vi "Pfeiffer-RVC300.ProcCases.vi"(0 "i ref in":refnum<vi>, 1 "selector":string, 2 "Data":T1, 3 "call cluster":T2={"Object"="", "Selector"="", "CallType"=enum."synchronous", "Async Object"="", "Async Selector"="", "Data Descriptor"="", "Data"=[], "Error #"=0, "Expire"=0}, 5 "error in (no error)":errorcluster) -> (14 "i ref out":refnum<vi>, 17 "answer cluster":T2={"Object"="", "Selector"="", "CallType"=enum."synchronous", "Async Object"="", "Async Selector"="", "Data Descriptor"="", "Data"=[], "Error #"=0, "Expire"=0}, 19 "error out":errorcluster)   [LabVIEW 2014, in "Pfeiffer-RVC300.lvlib"]
doc: "This method is called by a process from within the default case in the event loop. The methods of a class that are linked to events will be called from THIS method. Add your code here."
uses:
  Pfeiffer-RVC300.lvlib
  CS_Core/CSSystem/CoreDefs/CoreDefs.call_type.ctl
  CS_Core/BaseProcess/BaseProcess.descriptor string definition.ctl
  CS_Core/CSSystem/CoreDefs/CoreDefs.rawDataType.ctl
  CS_Core/CSSystem/CoreLib/CoreLib.byte array 2 double.vi
  CS_Core/CSSystem/CoreLib/CoreLib.double 2 byte array.vi
  CS_Core/CSSystem/CoreLib/CoreLib.string 2 byte array.vi
  CS_Core/CSSystem/CoreLib/CoreLib.byte array 2 int.vi
  CS_Core/CSSystem/CoreLib/CoreLib.lvlib
  CS_Core/BaseProcess/BaseProcess.lvlib
  CS_Core/CSApplicationBaseClasses/DeviceBase/DeviceBase.lvlib
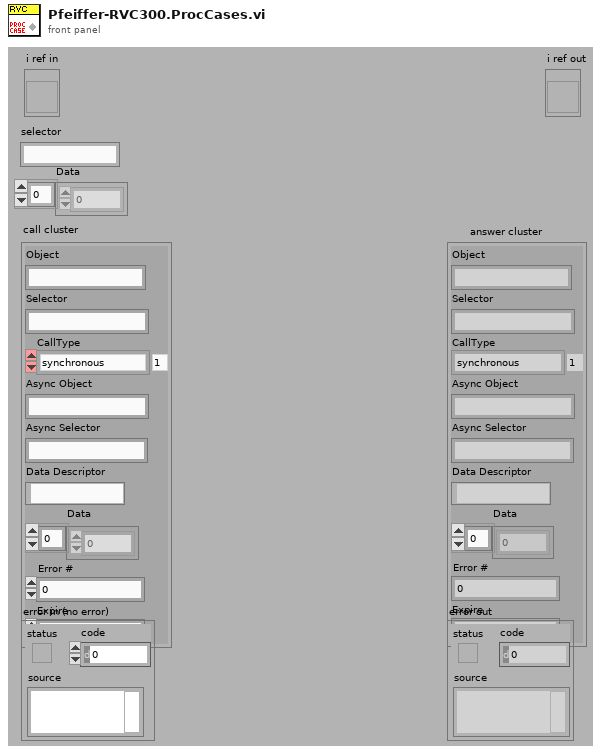
[diagram p1: front panel]
types:
  T1 = typedef "CoreDefs.rawDataType.ctl" = i8[]
  T2 = typedef "CoreDefs.call_type.ctl" = cluster{"Object":string, "Selector":string, "CallType":enum16{"simple", "synchronous", "asynchronous"}, "Async Object":string, "Async Selector":string, "Data Descriptor":T3, "Data":T1, "Error #":i32, "Expire":u32}
  T3 = typedef "BaseProcess.lvlib/BaseProcess.descriptor string definition.ctl" = string
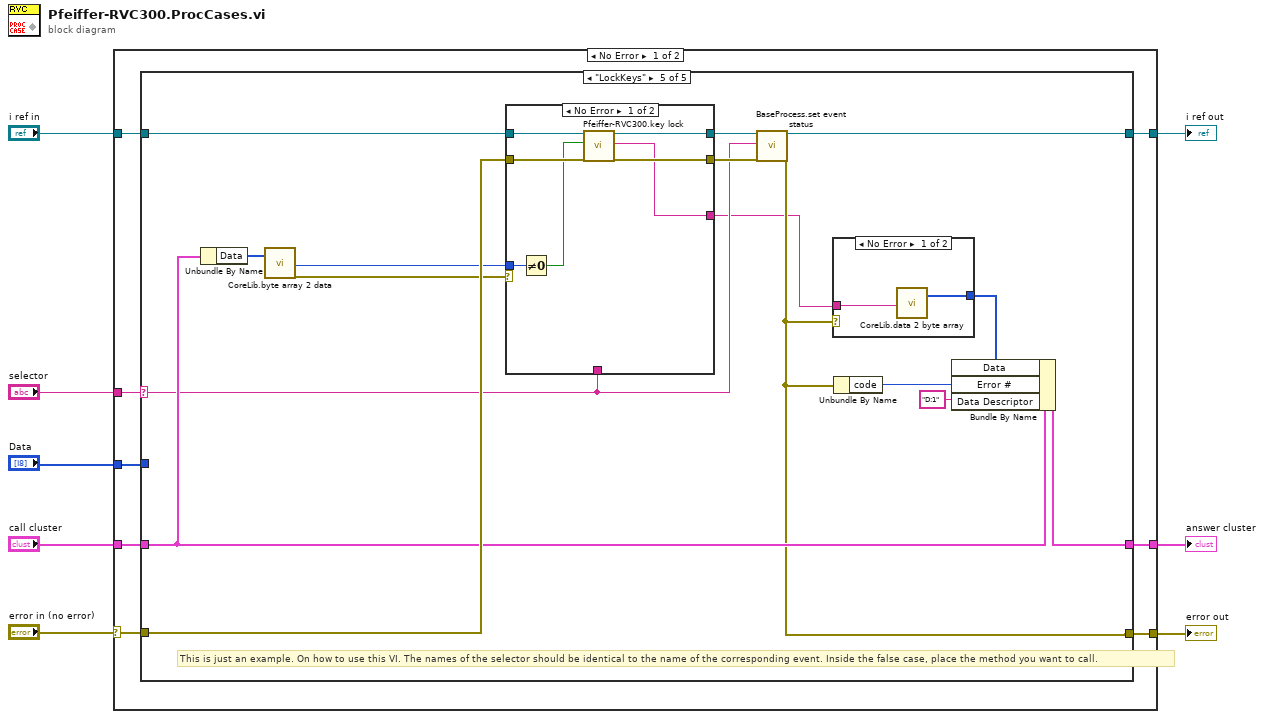
[diagram p0: block diagram]
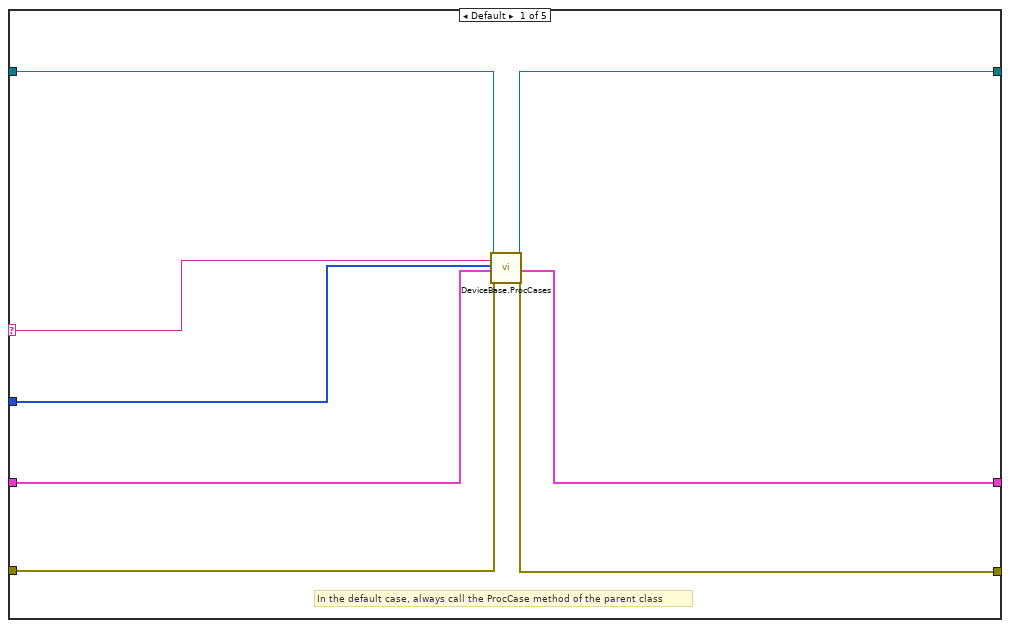
[diagram p2: hidden frame]
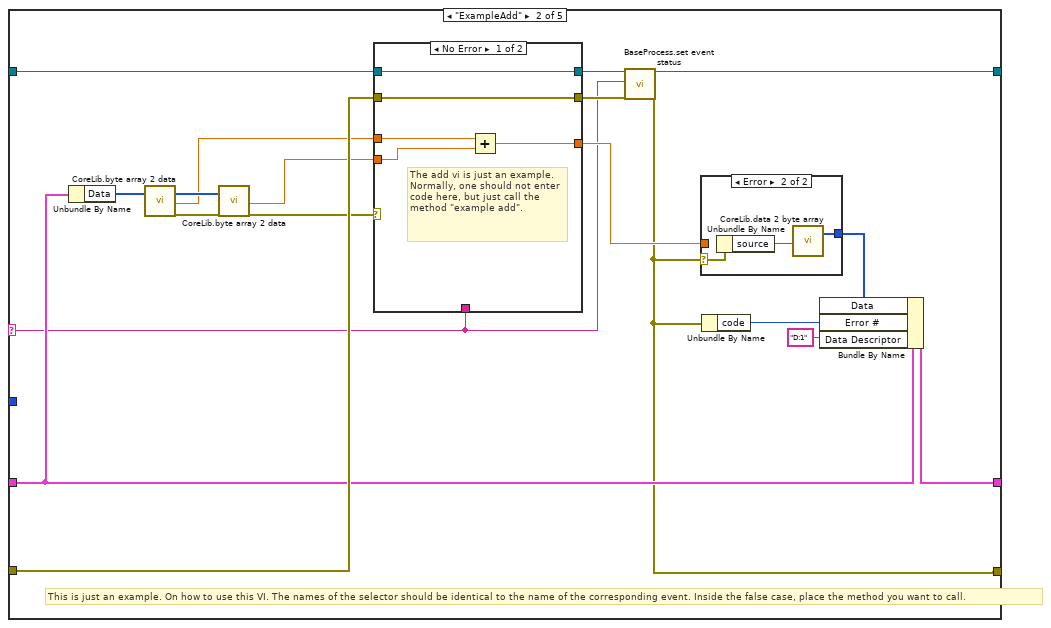
[diagram p3: hidden frame]
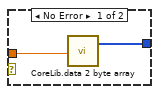
[diagram p4: hidden frame]
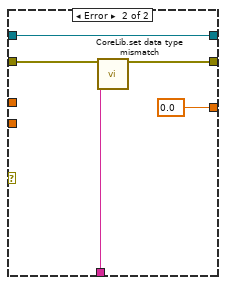
[diagram p5: hidden frame]
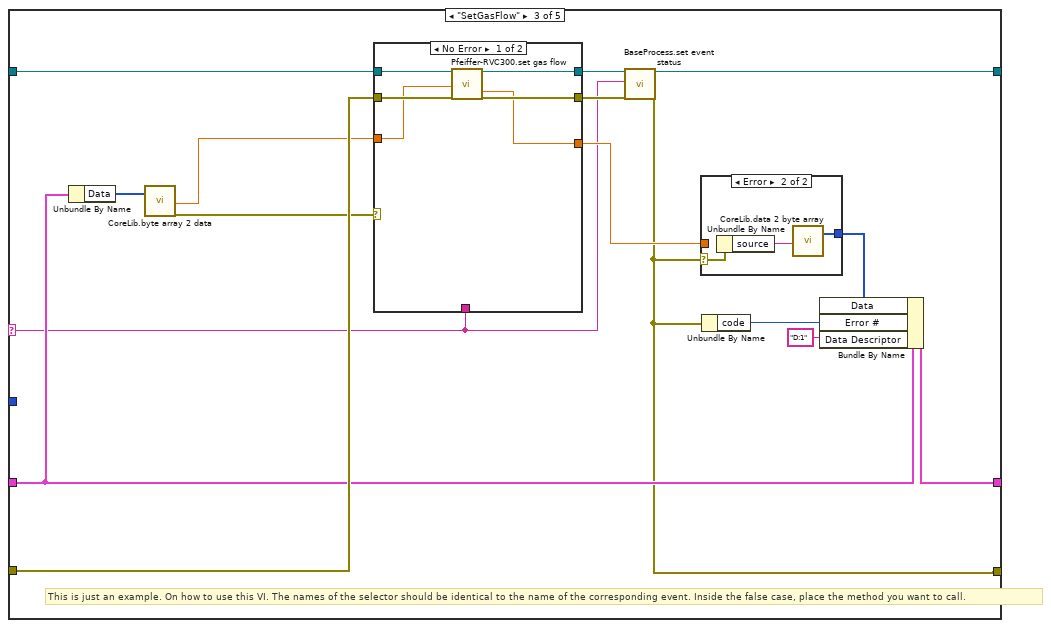
[diagram p6: hidden frame]
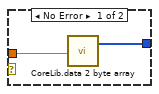
[diagram p7: hidden frame]
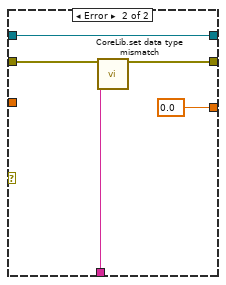
[diagram p8: hidden frame]
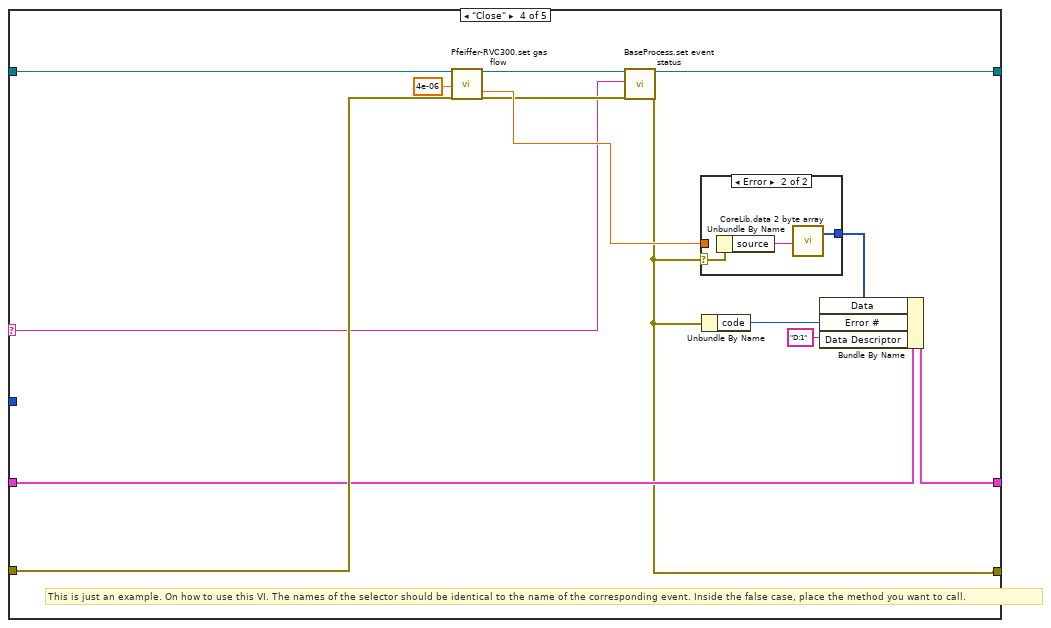
[diagram p9: hidden frame]
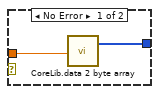
[diagram p10: hidden frame]
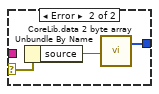
[diagram p11: hidden frame]
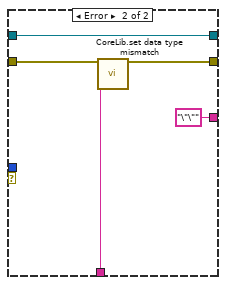
[diagram p12: hidden frame]
diagram:
  n1 = case shown="No Error" "error in (no error)" {
    selector: "error in (no error)" -> [w9 w143]
    tunnel: "selector" -> [w16 _]
    tunnel: [w15 w144] -> w7
    tunnel: "Data" -> [w14 _]
    tunnel: "call cluster" -> [w13 w144]
    tunnel: "i ref in" -> [w12 w145]
    tunnel: [w11 w145] -> w3
    tunnel: [w10 w143] -> w2
    frame No Error {
      n2 = case shown="\"LockKeys\"" w16 {
        selector: w16 -> [w19 w33 w64 w94 w116]
        tunnel: w14 -> [w17 _ _ _ _]
        tunnel: w12 -> [w18 w43 w74 w104 w125]
        tunnel: [w24 w32 w63 w93 w115] -> w11
        tunnel: w13 -> [w20 w39 w70 w100 w122]
        tunnel: [w21 w38 w69 w99 w121] -> w15
        tunnel: w9 -> [w23 w42 w73 w103 w124]
        tunnel: [w22 w34 w65 w95 w117] -> w10
        frame Default {
          # "In the default case, always call the ProcCase method of the parent class"
          n3 = call "DeviceBase.ProcCases.vi"("i ref in"=w18, "selector"=w19, "Data"=w17, "call cluster"=w20, "error in (no error)"=w23) -> ("i ref out"=w24:refnum<vi>, "answer cluster"=w21:T2, "error out"=w22:errorcluster)  [unwired: 12 in]
        }
        frame "ExampleAdd" {
          # "This is just an example. On how to use this VI. The names of the selector should be identical to the name of the corresponding event. Inside the false case, place the method you want to call."
          n4 = Unbundle By Name(w39) -> ("Data"=w30:T1)
          n5 = call-poly "CoreLib.byte array 2 data.vi"("byteArray"=w30) -> ("byteArray out"=w28:T1, "d64"=w26:dbl, "error out"=w29:errorcluster)  [unwired: 16 in]
          n6 = call-poly "CoreLib.byte array 2 data.vi"("byteArray"=w28, "error in (no error)"=w29) -> ("d64"=w25:dbl, "error out"=w27:errorcluster)  [unwired: 15 in, 1 out]
          n7 = case shown="No Error" w27 {
            tunnel: [w50 w58] -> w36
            tunnel: w43 -> [w50 w58]
            tunnel: w42 -> [w51 w57]
            tunnel: [w51 w56] -> w35
            tunnel: w25 -> [w53 _]
            tunnel: [w52 0.0] -> w41
            tunnel: w33 -> [_ w54]
            tunnel: w26 -> [w49 _]
            frame No Error {
              # "The add vi is just an example. Normally, one should not enter code here, but just call the method \"example add\"."
              n8 = Add(x=w49, y=w53) -> (x+y=w52:dbl)
            }
            frame Error {
              n9 = call "CoreLib.set data type mismatch.vi"("error in (no error)"=w57, "error source"=w54) -> ("error out"=w56:errorcluster)  [unwired: 17 in]
            }
          }
          n10 = call "BaseProcess.set event status.vi"("i ref in"=w36, "EventStatus"=w33, "error in (no error)"=w35) -> ("i ref out"=w32:refnum<vi>, "error out"=w34:errorcluster)  [unwired: 14 in, 1 out]
          n11 = case shown="Error" w34 {
            selector: w34 -> [_ w48]
            tunnel: [w44 w47] -> w37
            tunnel: w41 -> [w45 _]
            frame No Error {
              n12 = call-poly "CoreLib.data 2 byte array.vi"("f64"=w45) -> ("byteArray out"=w44:T1)  [unwired: 18 in]
            }
            frame Error {
              n13 = Unbundle By Name(w48) -> ("source"=w46:string)
              n14 = call-poly "CoreLib.data 2 byte array.vi"("string"=w46) -> ("byteArray out"=w47:T1)  [unwired: 18 in]
            }
          }
          n15 = Unbundle By Name(w34) -> ("code"=w40:i32)
          n16 = Bundle By Name(cluster=w39, "Data"=w37, "Error #"=w40, "Data Descriptor"="D:1") -> (w38:T2)
        }
        frame "SetGasFlow" {
          # "This is just an example. On how to use this VI. The names of the selector should be identical to the name of the corresponding event. Inside the false case, place the method you want to call."
          n17 = Unbundle By Name(w70) -> ("Data"=w61:T1)
          n18 = call-poly "CoreLib.byte array 2 data.vi"("byteArray"=w61) -> ("d64"=w60:dbl, "error out"=w59:errorcluster)  [unwired: 16 in, 1 out]
          n19 = case shown="No Error" w59 {
            tunnel: [w84 w90] -> w67
            tunnel: w74 -> [w85 w90]
            tunnel: w73 -> [w83 w89]
            tunnel: [w82 w88] -> w66
            tunnel: [w81 0.0] -> w72
            tunnel: w64 -> [_ w86]
            tunnel: w60 -> [w80 _]
            frame No Error {
              n20 = call "Pfeiffer-RVC300.set gas flow.vi"("i ref in"=w85, "gas_flow"=w80, "error in (no error)"=w83) -> ("i ref out"=w84:refnum<vi>, "gas_flow_out"=w81:dbl, "error out"=w82:errorcluster)  [unwired: 14 in]
            }
            frame Error {
              n21 = call "CoreLib.set data type mismatch.vi"("error in (no error)"=w89, "error source"=w86) -> ("error out"=w88:errorcluster)  [unwired: 17 in]
            }
          }
          n22 = call "BaseProcess.set event status.vi"("i ref in"=w67, "EventStatus"=w64, "error in (no error)"=w66) -> ("i ref out"=w63:refnum<vi>, "error out"=w65:errorcluster)  [unwired: 14 in, 1 out]
          n23 = case shown="Error" w65 {
            selector: w65 -> [_ w79]
            tunnel: [w75 w78] -> w68
            tunnel: w72 -> [w76 _]
            frame No Error {
              n24 = call-poly "CoreLib.data 2 byte array.vi"("f64"=w76) -> ("byteArray out"=w75:T1)  [unwired: 18 in]
            }
            frame Error {
              n25 = Unbundle By Name(w79) -> ("source"=w77:string)
              n26 = call-poly "CoreLib.data 2 byte array.vi"("string"=w77) -> ("byteArray out"=w78:T1)  [unwired: 18 in]
            }
          }
          n27 = Unbundle By Name(w65) -> ("code"=w71:i32)
          n28 = Bundle By Name(cluster=w70, "Data"=w68, "Error #"=w71, "Data Descriptor"="D:1") -> (w69:T2)
        }
        frame "Close" {
          # "This is just an example. On how to use this VI. The names of the selector should be identical to the name of the corresponding event. Inside the false case, place the method you want to call."
          n29 = call "Pfeiffer-RVC300.set gas flow.vi"("i ref in"=w104, "gas_flow"=4e-06, "error in (no error)"=w103) -> ("i ref out"=w97:refnum<vi>, "gas_flow_out"=w102:dbl, "error out"=w96:errorcluster)  [unwired: 14 in]
          n30 = call "BaseProcess.set event status.vi"("i ref in"=w97, "EventStatus"=w94, "error in (no error)"=w96) -> ("i ref out"=w93:refnum<vi>, "error out"=w95:errorcluster)  [unwired: 14 in, 1 out]
          n31 = case shown="Error" w95 {
            selector: w95 -> [_ w109]
            tunnel: [w105 w108] -> w98
            tunnel: w102 -> [w106 _]
            frame No Error {
              n32 = call-poly "CoreLib.data 2 byte array.vi"("f64"=w106) -> ("byteArray out"=w105:T1)  [unwired: 18 in]
            }
            frame Error {
              n33 = Unbundle By Name(w109) -> ("source"=w107:string)
              n34 = call-poly "CoreLib.data 2 byte array.vi"("string"=w107) -> ("byteArray out"=w108:T1)  [unwired: 18 in]
            }
          }
          n35 = Unbundle By Name(w95) -> ("code"=w101:i32)
          n36 = Bundle By Name(cluster=w100, "Data"=w98, "Error #"=w101, "Data Descriptor"="D:1") -> (w99:T2)
        }
        frame "LockKeys" {
          # "This is just an example. On how to use this VI. The names of the selector should be identical to the name of the corresponding event. Inside the false case, place the method you want to call."
          n37 = Unbundle By Name(w122) -> ("Data"=w112:T1)
          n38 = call-poly "CoreLib.byte array 2 data.vi"("byteArray"=w112) -> ("i32"=w110:i32, "error out"=w111:errorcluster)  [unwired: 16 in, 1 out]
          n39 = case shown="No Error" w111 {
            tunnel: [w135 w142] -> w119
            tunnel: w125 -> [w136 w142]
            tunnel: w124 -> [w134 w141]
            tunnel: [w133 w140] -> w118
            tunnel: w116 -> [_ w139]
            tunnel: w110 -> [w137 _]
            tunnel: [w131 "\"\"" ("key_status")] -> w113
            frame No Error {
              n40 = Not Equal To 0?(x=w137) -> (x != 0?=w132:bool)
              n41 = call "Pfeiffer-RVC300.key lock.vi"("i ref in"=w136, "Lock?"=w132, "error in (no error)"=w134) -> ("i ref out"=w135:refnum<vi>, "key_status"=w131:string, "error out"=w133:errorcluster)  [unwired: 14 in]
            }
            frame Error {
              n42 = call "CoreLib.set data type mismatch.vi"("error in (no error)"=w141, "error source"=w139) -> ("error out"=w140:errorcluster)  [unwired: 17 in]
            }
          }
          n43 = call "BaseProcess.set event status.vi"("i ref in"=w119, "EventStatus"=w116, "error in (no error)"=w118) -> ("i ref out"=w115:refnum<vi>, "error out"=w117:errorcluster)  [unwired: 14 in, 1 out]
          n44 = case shown="No Error" w117 {
            selector: w117 -> [_ w130]
            tunnel: [w126 w129] -> w120
            tunnel: w113 -> [w127 _]
            frame No Error {
              n45 = call-poly "CoreLib.data 2 byte array.vi"("string"=w127) -> ("byteArray out"=w126:T1)  [unwired: 18 in]
            }
            frame Error {
              n46 = Unbundle By Name(w130) -> ("source"=w128:string)
              n47 = call-poly "CoreLib.data 2 byte array.vi"("string"=w128) -> ("byteArray out"=w129:T1)  [unwired: 18 in]
            }
          }
          n48 = Unbundle By Name(w117) -> ("code"=w123:i32)
          n49 = Bundle By Name(cluster=w122, "Data"=w120, "Error #"=w123, "Data Descriptor"="D:1") -> (w121:T2)
        }
      }
    }
    frame Error {
    }
  }
  "answer cluster" <- w7
  "i ref out" <- w3
  "error out" <- w2
